vi "Add BC Command (RT-BC).vi"(6 "messageBufferIDRef(-1)":i32=-1, 7 "monitor(F)":bool, 8 "error in":errorcluster, 9 "Message Command Configuration":T1, 10 "name":string, 11 "BusController in":refnum<k24>) -> (0 "error out":errorcluster, 2 "Message Command ID out":i32, 3 "BusController out":refnum<k24>)   [LabVIEW 2020, in "Ballard_1553_Hardware_ni.lvlib"]
uses:
  Ballard_1553_Hardware_ni.lvlib
  C:/Users/Administrator/Desktop/GIT/Ballard-MIL-STD-1553-Custom-Device/Source/System Explorer/SubVIs/Parse XML Ballard/1.2/BTIXML_SerDes.dll
  Ballard-MIL-STD-1553-Custom-Device/Source/System Explorer/SubVIs/Parse XML Ballard/1.2/BTIXML_SerDes.dll
  _typedefs/MessageCommand_BCRT_type.ctl
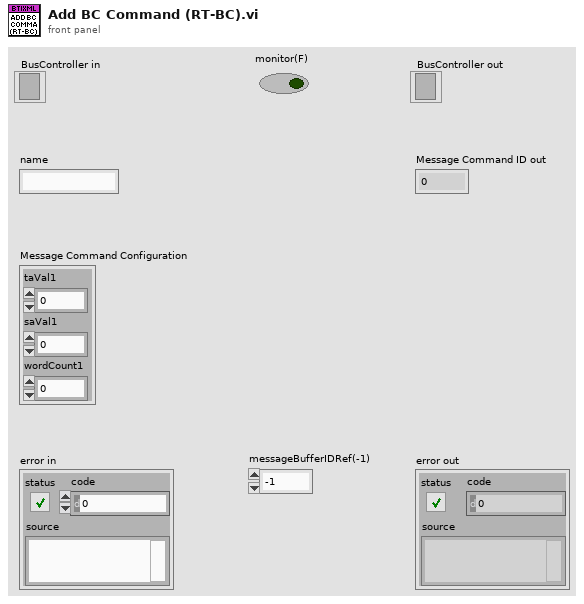
[diagram p1: front panel]
types:
  T1 = typedef "Ballard_1553_Hardware_ni.lvlib/MessageCommand_BCRT_type.ctl" = cluster{"taVal1":i8, "saVal1":i8, "wordCount1":i8}
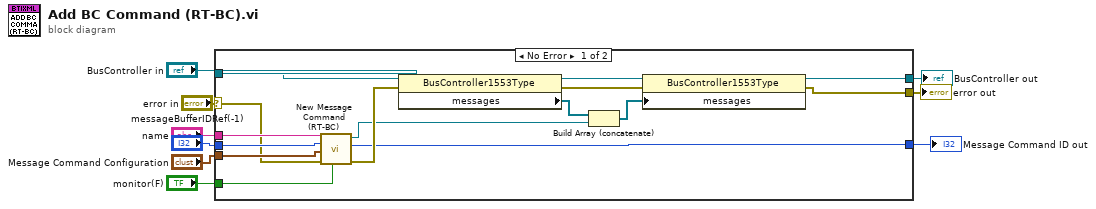
[diagram p0: block diagram]
diagram:
  n1 = case shown="No Error" "error in" {
    selector: "error in" -> [w11 w25]
    tunnel: [w21 w25] -> w9
    tunnel: [w22 w26] -> w8
    tunnel: "BusController in" -> [w24 w26]
    tunnel: [w16 _] -> w5
    tunnel: "name" -> [w14 _]
    tunnel: "messageBufferIDRef(-1)" -> [w13 _]
    tunnel: "Message Command Configuration" -> [w12 _]
    tunnel: "monitor(F)" -> [w10 _]
    frame No Error {
      n2 = call "New Message Command (RT-BC).vi"("monitor(F)"=w10, "error in"=w11, "Message Command Configuration"=w12, "messageBufferIDRef"=w13, "name"=w14) -> ("error out"=w18:errorcluster, "Message Command ID out"=w16:i32, "new message command"=w15:refnum<k24>)  [unwired: 4 in]
      n3 = property class="BusController1553Type"(reference=w24, error in=w18) -> (reference out=w23:refnum<k24>, error out=w20:errorcluster, "messages"=w19:refnum<k24>[])
      n4 = Build Array (concatenate)(w19, w15) -> (w17:refnum<k24>[])
      n5 = property class="BusController1553Type"(reference=w23, error in=w20, "messages"=w17) -> (reference out=w22:refnum<k24>, error out=w21:errorcluster)
    }
    frame Error {
    }
  }
  "error out" <- w9
  "BusController out" <- w8
  "Message Command ID out" <- w5
